vi "run.vi"(8 "error in (no error)":errorcluster, 10 "test":refnum<class>, 11 "TextTestRunner in":refnum<class "TestRunner.lvclass">) -> (0 "error out":errorcluster, 2 "TestResult out":refnum<class "TestResult.lvclass">, 3 "TextTestRunner out":refnum<class "TestRunner.lvclass">)   [LabVIEW 2019, in "TestRunner.lvclass"]
uses:
  TestRunner.lvclass
  TestResult/TestResult.lvclass
  TestRunner.lvclass/TestRunner.ctl
  TestSuite/TestSuite.lvclass
  TestCase/TestCase.lvclass
  Libraries/VITesterUtilities.lvlib
panel:
  # "JKI VI Tester for LabVIEW\nhttp://jkisoft.com/vi-tester\nCopyright (C) 2007-2009, JKI <info@jkisoft.com>\nALL RIGHTS RESERVED"
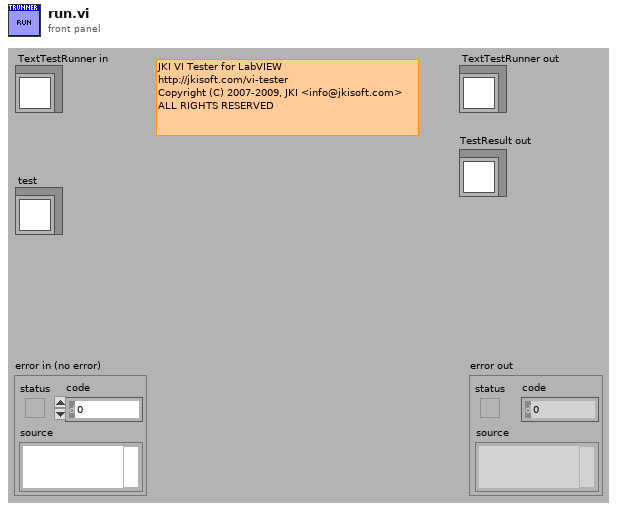
[diagram p1: front panel]
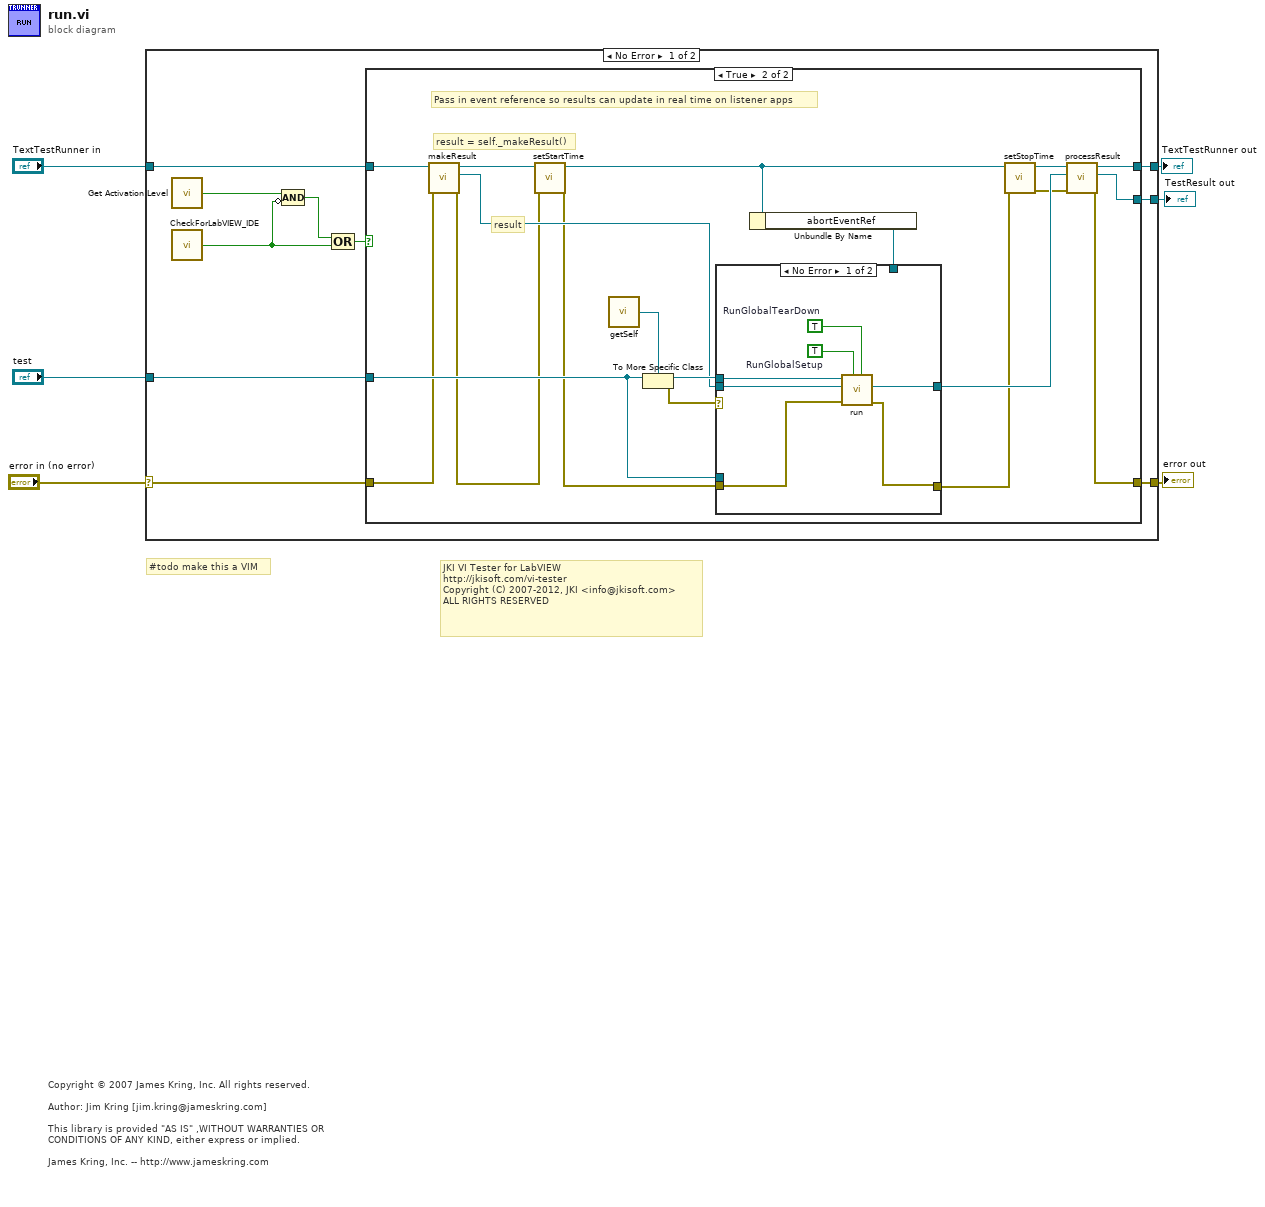
[diagram p0: block diagram]
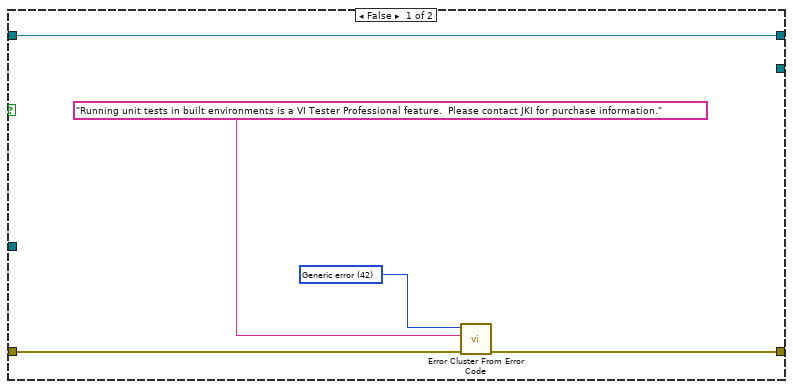
[diagram p2: hidden frame]
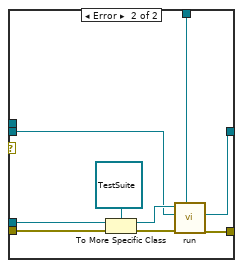
[diagram p3: hidden frame]
diagram:
  # "#todo make this a VIM"
  # "JKI VI Tester for LabVIEW\nhttp://jkisoft.com/vi-tester\nCopyright (C) 2007-2012, JKI <info@jkisoft.com>\nALL RIGHTS RESERVED"
  # "Copyright © 2007 James Kring, Inc. All rights reserved.\n\nAuthor: Jim Kring [jim.kring@jameskring.com]\n\nThis library is provided \"AS IS\" ,WITHOUT WARRANTIES OR \nCONDITIONS OF ANY KIND, either express or implied.\n\nJames Kring, Inc. -- http://www.jameskring.com"
  n1 = case shown="No Error" "error in (no error)" {
    selector: "error in (no error)" -> [w14 w58]
    tunnel: [w13 w58] -> w5
    tunnel: [w12 w57] -> w3
    tunnel: "TextTestRunner in" -> [w16 w57]
    tunnel: "test" -> [w15 _]
    tunnel: [w11 _] -> w1
    frame No Error {
      n2 = call "Get Activation Level.vi"() -> ("Valid Professional Version"=w8:bool)
      n3 = call "CheckForLabVIEW_IDE.vi"() -> ("LabVIEW IDE"=w7:bool)
      n4 = Compound Arithmetic op=AND(w8, invert w7) -> (w10:bool)
      n5 = Compound Arithmetic op=OR(w10, w7) -> (w9:bool)
      n6 = case shown="True" w9 {
        tunnel: w16 -> [w21 w40]
        tunnel: w15 -> [_ w37]
        tunnel: w14 -> [w20 w36]
        tunnel: [w19 w31] -> w13
        tunnel: [w21 w30] -> w12
        tunnel: [_ w23] -> w11
        frame False {
          w18 = 42 items=["No error", "Argument error", "Memory is full", "Out of zone", "End of file", "File already open", "Generic file I/O error", "File not found", "File permission error", "Disk is full", "Duplicate path", "Too many files open", "System feature not enabled", "Resource file not found", "Cannot add resource", "Resource not found", "Image not found", "Image memory error", "Pen does not exist", "Config type invalid", "Config token not found", "Config parse error", "Config memory error", "Bad external code format", "Bad external code offset", "External code not present", "Null window", "Destroy window error", "Null menu", "Print aborted", "Bad print record", "Print driver error", "Windows error during printing", "Memory error during printing", "Print dialog error", "Generic print error", "Invalid device refnum", "Device not found", "Device parameter error", "Device unit error", "Cannot open device", "Device call aborted", "Generic error", "Cancelled by user", "Object ID too low", "Object ID too high", "Object not in heap", "Unknown heap", "Unknown object (invalid DefProc)", "Unknown object (DefProc not in table)", "Message out of range", "Invalid (null) method", "Unknown message", "Manager call not supported", "Bad address", "Network operation in progress", "Network operation timed out", "Connection is busy", "Network attribute not supported", "Network error", "Address in use", "System out of memory", "Connection aborted", "Connection refused", "Not connected", "Already connected", "Connection closed", "Initialization error (interapplication manager)", "Bad occurrence", "Wait on unbound occurrence handler", "Occurrence queue overflow", "Datalog type conflict", "Unused", "Unrecognized type (interapplication manager)", "Memory corrupt", "Failed to make temporary DLL", "Old CIN version", "Drag socket not found", "Failed to load drop-object", "Failed to register OLE object", "Failed to release OLE object", "Format specifier type mismatch", "Unknown format specifier", "Too few format specifiers", "Too many format specifiers", "Scan failed", "Newer CIN version", "Error converting to variant", "Runtime menu error", "Password tampered", "Variant attribute not found", "Incompatible variant data type", "Event data is not available", "Event Store is not present", "Occurrence is not found", "Event Queue is not created", "Event info is not available", "Refnum passed is NULL", "Error retrieving Class GUID", "Error retrieving CoClass GUID", "Error retrieving TypeLib GUID.", "Bad built application magic bytes.", "Specific driver is different from the specific driver associated with the Logical Name.", "There is no session opened to the class driver.", "Max Error", "MAX - Error with config objects", "MAX - Error loading configuration", "MAX - Group not supported"]
          n7 = call <vilib>:"Error Cluster From Error Code.vi"("error in (no error)"=w20, "error message (\"\")"="Running unit tests in built environments is a VI Tester Professional feature.  Please contact JKI for purchase information.", "error code (0)"=w18) -> ("error out"=w19:errorcluster)  [unwired: 6 in]
        }
        frame True {
          # "Pass in event reference so results can update in real time on listener apps"
          # "result"
          # "result = self._makeResult()"
          n8 = call-dynamic "makeResult.vi"("error in (no error)"=w36, "TextTestRunner in"=w40) -> ("error out"=w32:errorcluster, "TestResult"=w34:refnum<class "TestResult.lvclass">, "TextTestRunner out"=w28:refnum<class "TestRunner.lvclass">)  [unwired: 7 in]
          n9 = call "setStartTime.vi"("error in"=w32, "TestRunner in"=w28) -> ("error out"=w33:errorcluster, "TestRunner out"=w26:refnum<class "TestRunner.lvclass">)  [unwired: 8 in]
          n10 = call "getSelf.vi"() -> ("TestCase.lvclass"=w22:refnum<class "TestCase.lvclass">)
          n11 = To More Specific Class(target class=w22, reference=w37) -> (specific class reference=w39:refnum<class "TestCase.lvclass">, error out=w38:errorcluster)  [unwired: 1 in]
          n12 = Unbundle By Name(w26) -> ("abortEventRef"=w29:refnum<user-event>)
          n13 = case shown="No Error" w38 {
            tunnel: w39 -> [w45 _]
            tunnel: w34 -> [w46 w50]
            tunnel: w37 -> [_ w56]
            tunnel: w33 -> [w42 w52]
            tunnel: [w41 w53] -> w27
            tunnel: [w47 w49] -> w35
            tunnel: w29 -> [_ w48]
            frame No Error {
              w43 = TRUE  # RunGlobalTearDown
              w44 = TRUE  # RunGlobalSetup
              n14 = call "run.vi"("RunGlobalTearDown"=w43, "RunGlobalSetup"=w44, "error in (no error)"=w42, "TestResult in (None: Create New)"=w46, "TestCase in"=w45) -> ("error out"=w41:errorcluster, "TestResult out"=w47:refnum<class "TestResult.lvclass">)  [unwired: 4 in, 1 out]
            }
            frame Error {
              n15 = To More Specific Class(target class=refnum<class "TestSuite.lvclass"> refnum ("reference in"), reference=w56, error in=w52) -> (specific class reference=w54:refnum<class "TestSuite.lvclass">, error out=w51:errorcluster)
              n16 = call "run.vi"("abortEvent"=w48, "error in (no error)"=w51, "TestResult in"=w50, "TestSuite in"=w54) -> ("error out"=w53:errorcluster, "TestResult out"=w49:refnum<class "TestResult.lvclass">)  [unwired: 5 in, 1 out]
            }
          }
          n17 = call "setStopTime.vi"("error in"=w27, "TestRunner in"=w26) -> ("error out"=w25:errorcluster, "TestRunner out"=w24:refnum<class "TestRunner.lvclass">)  [unwired: 8 in]
          n18 = call-dynamic "processResult.vi"("error in"=w25, "TestResult in"=w35, "TestRunner in"=w24) -> ("error out"=w31:errorcluster, "TestResult out"=w23:refnum<class "TestResult.lvclass">, "TestRunner out"=w30:refnum<class "TestRunner.lvclass">)  [unwired: 6 in]
        }
      }
    }
    frame Error {
    }
  }
  "error out" <- w5
  "TextTestRunner out" <- w3
  "TestResult out" <- w1
